vi "MTMount_putSample_EncoderEIB.vi"(8 "error in (no error)":errorcluster, 11 "Encoder_EIB_Ctl":T1) -> (0 "error out":errorcluster, 2 "function return":i32, 3 "Encoder_EIB_Ctl out":T1)   [LabVIEW 2018, in "SALLV_MTMount.lvlib"]
doc: "int MTMount_shm_putSample_Encoder_EIBLV(MTMount_Encoder_EIBLV *Encoder_EIB_Ctl );"
uses:
  SALLV_MTMount.lvlib
  DataTypes/Encoder_EIB.ctl
  SALLV_MTMount.so
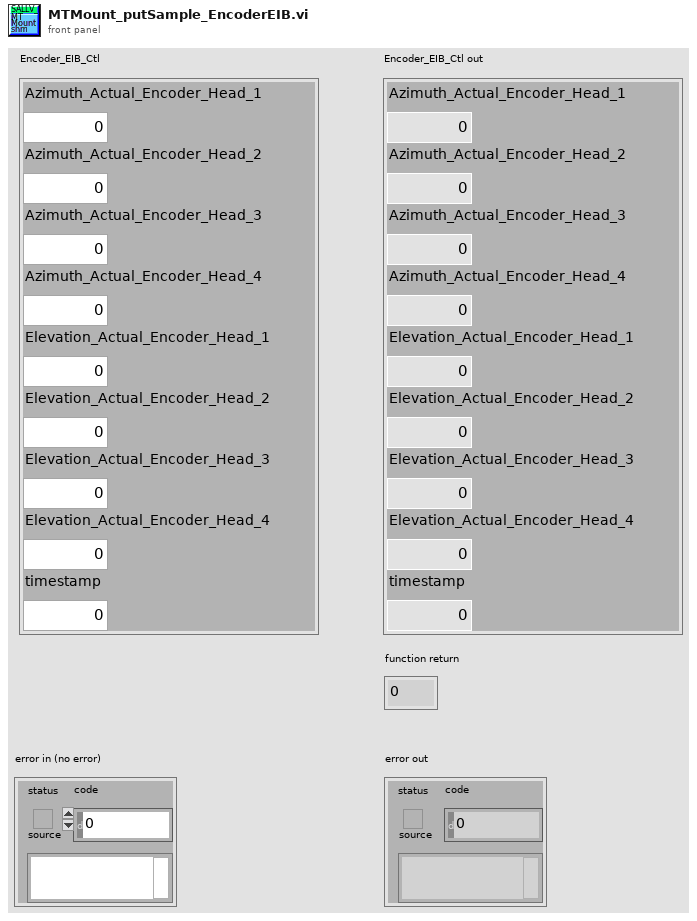
[diagram p1: front panel]
types:
  T1 = typedef "SALLV_MTMount.lvlib/Encoder_EIB.ctl" = cluster{"Azimuth_Actual_Encoder_Head_1":u32, "Azimuth_Actual_Encoder_Head_2":u32, "Azimuth_Actual_Encoder_Head_3":u32, "Azimuth_Actual_Encoder_Head_4":u32, "Elevation_Actual_Encoder_Head_1":u32, "Elevation_Actual_Encoder_Head_2":u32, "Elevation_Actual_Encoder_Head_3":u32, "Elevation_Actual_Encoder_Head_4":u32, "timestamp":dbl}
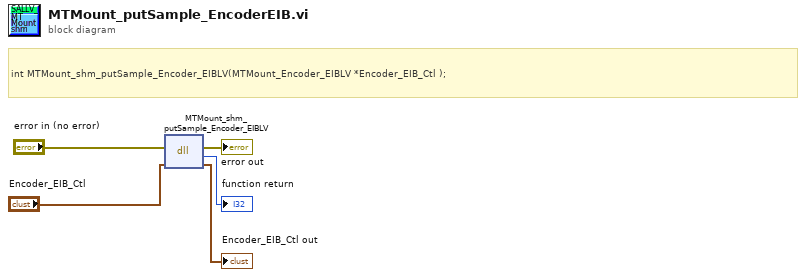
[diagram p0: block diagram]
diagram:
  # "int MTMount_shm_putSample_Encoder_EIBLV(MTMount_Encoder_EIBLV *Encoder_EIB_Ctl );"
  n1 = dll-call lib="home/ttsai/Document/salApiMTMount/SALLV_MTMount/SALLV_MTMount.*" fn="MTMount_shm_putSample_Encoder_EIBLV"(error in="error in (no error)", "Encoder_EIB_Ctl"="Encoder_EIB_Ctl") -> (error out=→"error out":errorcluster, →"function return":i32, "Encoder_EIB_Ctl"=→"Encoder_EIB_Ctl out":T1)  [unwired: 2 in, 1 out]
